vi "pp2_overwriteSI_Stim.vi"(10 "New Stim":bool=TRUE, 11 "State Info In":T1={"Curr  tr"=0, "Curr (ms)"=0, "Cum (ms)"=0, "Run loop diff"=0, "Tone countdown (ms)"=0, "Countdown (ms)"=0, "Curr type"=0, "Curr State"=enum."0 Habituation", "Prev State"=enum."0 Habituation", "Null"=FALSE, "Sw1"=FALSE, "Tone\nGate"=FALSE, "Sw2"=FALSE, "Stim"=FALSE, "Current DAQ DO Int"=0, "Current Loaded Trial"={"Trial Type Number"=1, "Trial Type"=enum."GO", "Trial Weight"=100, "Shock (mA)"=0.3, "Duration (ms)"=0.25, "Type"=enum."04 FM Sweep", "Stim P2"=4000.0, "Stim P3"=0.0, "Stim P4"=0.0, "Stim P1"=2000.0}, "Next Trial"={"Trial Type Number"=1, "Trial Type"=enum."GO", "Trial Weight"=100, "Shock (mA)"=0.3, "Duration (ms)"=0.25, "Type"=enum."04 FM Sweep", "Stim P2"=4000.0, "Stim P3"=0.0, "Stim P4"=0.0, "Stim P1"=2000.0}} {"Current DAQ DO Int" format="%b"; "Next Trial"."Shock (mA)" min=-1.0 max=5.0; "Next Trial"."Trial Weight" step=1; "Next Trial"."Duration (ms)" min=0.0 max=1.0; "Next Trial"."Trial Type Number" min=1 max=256 step=1; "Current Loaded Trial"."Shock (mA)" min=-1.0 max=5.0; "Current Loaded Trial"."Trial Weight" step=1; "Current Loaded Trial"."Duration (ms)" min=0.0 max=1.0; "Current Loaded Trial"."Trial Type Number" min=1 max=256 step=1; "Curr type" format="%#.6f"}) -> (3 "State Info Out":T1={"Curr  tr"=0, "Curr (ms)"=0, "Cum (ms)"=0, "Run loop diff"=0, "Tone countdown (ms)"=0, "Countdown (ms)"=0, "Curr type"=0, "Curr State"=enum."0 Habituation", "Prev State"=enum."0 Habituation", "Null"=FALSE, "Sw1"=FALSE, "Tone\nGate"=FALSE, "Sw2"=FALSE, "Stim"=FALSE, "Current DAQ DO Int"=0, "Current Loaded Trial"={"Trial Type Number"=1, "Trial Type"=enum."GO", "Trial Weight"=100, "Shock (mA)"=0.3, "Duration (ms)"=0.25, "Type"=enum."04 FM Sweep", "Stim P2"=4000.0, "Stim P3"=0.0, "Stim P4"=0.0, "Stim P1"=2000.0}, "Next Trial"={"Trial Type Number"=1, "Trial Type"=enum."GO", "Trial Weight"=100, "Shock (mA)"=0.3, "Duration (ms)"=0.25, "Type"=enum."04 FM Sweep", "Stim P2"=4000.0, "Stim P3"=0.0, "Stim P4"=0.0, "Stim P1"=2000.0}} {"Current DAQ DO Int" format="%b"; "Next Trial"."Shock (mA)" min=-1.0 max=5.0; "Next Trial"."Trial Weight" step=1; "Next Trial"."Duration (ms)" min=0.0 max=1.0; "Next Trial"."Trial Type Number" min=1 max=256 step=1; "Current Loaded Trial"."Shock (mA)" min=-1.0 max=5.0; "Current Loaded Trial"."Trial Weight" step=1; "Current Loaded Trial"."Duration (ms)" min=0.0 max=1.0; "Current Loaded Trial"."Trial Type Number" min=1 max=256 step=1; "Curr type" format="%#.6f"})   [LabVIEW 2013]
uses:
  pp2_CTL_StateInfo.ctl
  pp2_CTL_State.ctl
  pp2_Trial.ctl
  pp2_CTL_TrialType.ctl
  labolabo2/waveforms/WFTypes.ctl
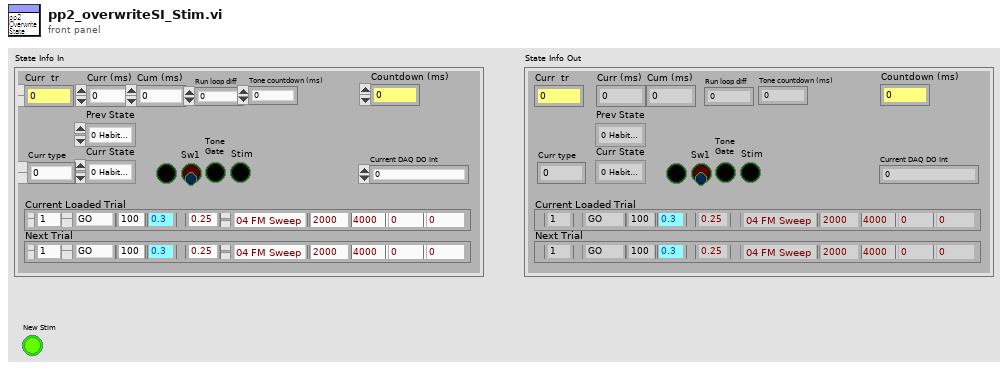
[diagram p1: front panel]
types:
  T1 = typedef "pp2_CTL_StateInfo.ctl" = cluster{"Curr  tr":u16, "Curr (ms)":i64, "Cum (ms)":i64, "Run loop diff":i64, "Tone countdown (ms)":i64, "Countdown (ms)":i64, "Curr type":u8, "Curr State":T2, "Prev State":T2, "Null":bool, "Sw1":bool, "Tone\nGate":bool, "Sw2":bool, "Stim":bool, "Current DAQ DO Int":u16, "Current Loaded Trial":T3, "Next Trial":T3}
  T2 = typedef "pp2_CTL_State.ctl" = enum8{"0 Habituation", "1 Load Trial", "2 Stay period", "3 Pre", "4 GO Trial", "5 GO Jumped", "6 GO Timeout", "7 NOGO Trial", "8 NOGO Jumped", "9 NOGO Timeout", "10 TEST Trial", "11 TEST Jumped", "12 TEST Timeout", "13 Intertrial Interval", "14 Done"}
  T3 = typedef "pp2_Trial.ctl" = cluster{"Trial Type Number":i16, "Trial Type":T4, "Trial Weight":u32, "Shock (mA)":dbl, "Duration (ms)":dbl, "Type":T5, "Stim P2":dbl, "Stim P3":dbl, "Stim P4":dbl, "Stim P1":dbl}
  T4 = typedef "pp2_CTL_TrialType.ctl" = enum16{"OFF", "GO", "NOGO", "TEST"}
  T5 = typedef "WFTypes.ctl" = enum16{"00 NULL", "01 DC", "02 Noise", "03 Pure Tone", "04 FM Sweep"}
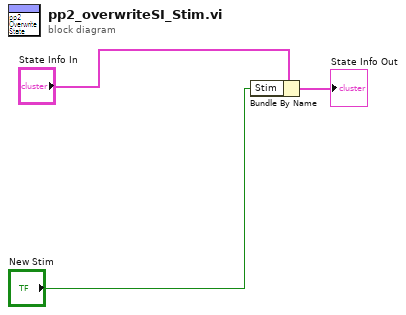
[diagram p0: block diagram]
diagram:
  n1 = Bundle By Name(cluster="State Info In", "Stim"="New Stim") -> (→"State Info Out":T1)
